vi "Build Project Build Spec.vi"(0 "NI Build Specification in":refnum<class "NI Build Specification_LV.lvclass">, 11 "error IO":errorcluster) -> (4 "NI Build Specification out":refnum<class "NI Build Specification_LV.lvclass">, 15 "error out":errorcluster)   [LabVIEW 2017, in "CL_G3_VIComponentBuilder.lvlib" / "NI Build Specification_LV.lvclass"]
doc: "Automates interactions with LabVIEW to build the specific Project Build specification. Builds all sub build specs in the <Anchor><Text>LabVIEW Project SubBuild Spec Order</Text><AnchorName>LabVIEW Project SubBuild Spec Order[]</AnchorName><PageName>NI Build Specification_LV Class Documentation</PageName><Space>TCS</Space></Anchor> and then builds the <Anchor><Text>Export's Build Spec Name</Text><AnchorName>Export's Build Spec Name</AnchorName><PageName>NI Build Specification_LV Class Documentation</PageName><Space>TCS</Space></Anchor>. <MustCallParent>The parent creates all sub exports and therefore must be called by the child of this class.</MustCallParent>"
uses:
  NI Build Specification_LV.lvclass
  NI Build Specification_LV.lvclass/NI Build Specification_LV.ctl
  Accessors/Read Export's Build Spec Name.vi
  Accessors/Read Target Name Containing Build Specs to Build.vi
  Accessors/Read LabVIEW Project SubBuild Spec Order.vi
  Accessors/Read Project Reference.vi
  <vilib>/AppBuilder/AB_API_Simple/Get Build Specification Version (project reference).vi
  <vilib>/AppBuilder/AB_API_Simple/Build (project reference).vi
  <vilib>/AppBuilder/AB_API_Simple/NI_App_Builder_API.lvlib
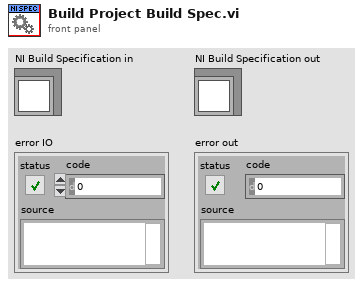
[diagram p1: front panel]
types:
  T1 = typedef "NI_App_Builder_API.lvlib/Build Specification Version.ctl" = cluster{"Major":u16, "Minor":u16, "Fix":u16, "Build":u16}
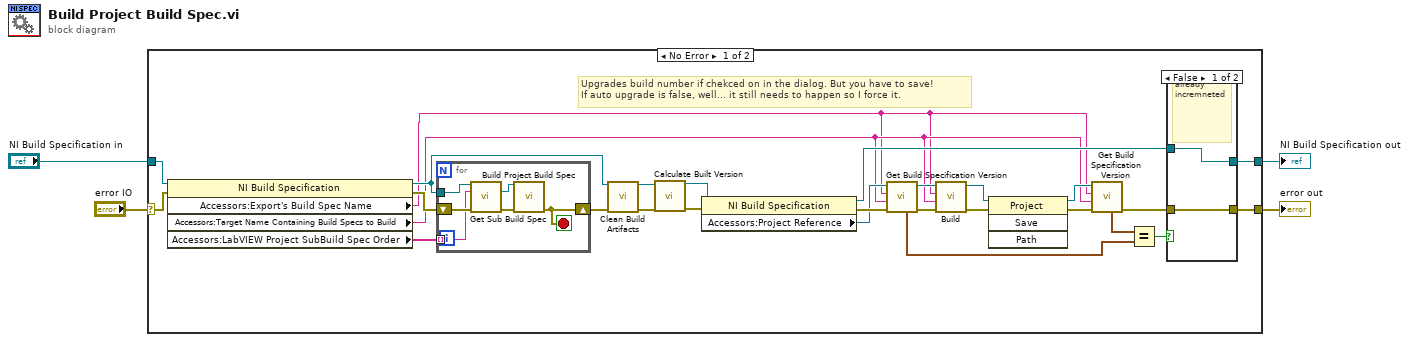
[diagram p0: block diagram]
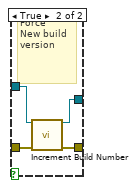
[diagram p2: hidden frame]
diagram:
  n1 = case shown="No Error" "error IO" {
    selector: "error IO" -> [w30 w45]
    tunnel: [w12 w45] -> w3
    tunnel: "NI Build Specification in" -> [w29 w44]
    tunnel: [w11 w44] -> w2
    frame No Error {
      # "Upgrades build number if chekced on in the dialog. But you have to save! \nIf auto upgrade is false, well... it still needs to happen so I force it."
      n2 = property class="NI Build Specification"(reference=w29, error in=w30) -> (reference out=w27:refnum<class "NI Build Specification_LV.lvclass">, error out=w31:errorcluster, "Accessors:Export's Build Spec Name"=w9:string, "Accessors:Target Name Containing Build Specs to Build"=w10:string, "Accessors:LabVIEW Project SubBuild Spec Order"=w28:string[])
      n3 = for {
        tunnel: w28 -> [w41] mode=indexing
        tunnel: w27 -> [w43]
        shift-right: [w38] -> w26
        shift-left: w31 -> [w42]
        stop <- w38 stop-if-true
        n4 = call "Get Sub Build Spec.vi"("NI Build Specification in"=w43, "Sub Build Spec Name"=w41, "error in (no error)"=w42) -> ("Sub Build Spec"=w39:refnum<class "NI Build Specification_LV.lvclass">, "error out"=w40:errorcluster)  [unwired: 9 in, 2 out]
        n5 = call-dynamic "Build Project Build Spec.vi"("NI Build Specification in"=w39, "error IO"=w40) -> ("error out"=w38:errorcluster)  [unwired: 12 in, 1 out]
      }
      n6 = call-dynamic "Clean Build Artifacts.vi"("NI Build Specification in"=w27, "error in (no error)"=w26) -> ("NI Build Specification out"=w8:refnum<class "NI Build Specification_LV.lvclass">, "error out"=w7:errorcluster)  [unwired: 12 in]
      n7 = call-dynamic "Calculate Built Version.vi"("NI Build Specification_LV in"=w8, "error in (no error)"=w7) -> ("NI Build Specification_LV out"=w5:refnum<class "NI Build Specification_LV.lvclass">, "error out"=w6:errorcluster)  [unwired: 12 in]
      n8 = property class="NI Build Specification"(reference=w5, error in=w6) -> (reference out=w15:refnum<class "NI Build Specification_LV.lvclass">, error out=w18:errorcluster, "Accessors:Project Reference"=w17:refnum<vi>)
      n9 = call-poly <vilib>:"Get Build Specification Version.vi"("error in (no error)"=w18, "Name of target (My Computer)"=w10, "Name of build specification"=w9, "Project reference"=w17) -> ("error out"=w25:errorcluster, "dup Project reference"=w14:refnum<vi>, "Build Specification Version"=w23:T1)  [unwired: 5 in]
      n10 = call-poly <vilib>:"Build.vi"("error in (no error)"=w25, "Name of target (My Computer)"=w10, "Name of build specification (if empty: build all)"=w9, "Project reference"=w14) -> ("error out"=w16:errorcluster, "project ref"=w13:refnum<vi>)  [unwired: 5 in, 1 out]
      n11 = invoke class="Project" method="Save"(reference=w13, error in=w16) -> (reference out=w19:refnum<vi>, error out=w20:errorcluster)  [unwired: 2 in, 2 out]
      n12 = call-poly <vilib>:"Get Build Specification Version.vi"("error in (no error)"=w20, "Name of target (My Computer)"=w10, "Name of build specification"=w9, "Project reference"=w19) -> ("error out"=w21:errorcluster, "Build Specification Version"=w24:T1)  [unwired: 5 in, 1 out]
      n13 = Equal?(x=w24, y=w23) -> (x = y?=w22:bool)
      n14 = case shown="False" w22 {
        tunnel: w15 -> [w32 w37]
        tunnel: w21 -> [w33 w36]
        tunnel: [w33 w35] -> w12
        tunnel: [w32 w34] -> w11
        frame False {
          # "already incremneted"
        }
        frame True {
          # "Force\nNew build version"
          n15 = call-dynamic "Increment Build Number.vi"("NI Build Specification in"=w37, "error in (no error)"=w36) -> ("NI Build Specification out"=w34:refnum<class "NI Build Specification_LV.lvclass">, "error out"=w35:errorcluster)  [unwired: 12 in]
        }
      }
    }
    frame Error {
    }
  }
  "NI Build Specification out" <- w2
  "error out" <- w3
